vi "StopFDC.vi"() -> ()   [LabVIEW 2013]
panel:
  in  "Positions Théoriques Moteurs":i32[](array[numeric])
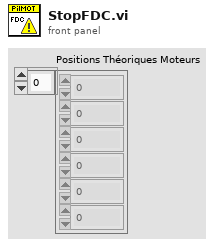
[diagram p1: front panel]
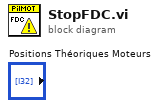
[diagram p0: block diagram]
diagram:
